vi "HEWH Build Draw Water States.vi"(8 "error in (no error)":errorcluster, 9 "Start Draw":bool, 10 "Full Cutout?":bool, 11 "Station":string) -> (0 "error out":errorcluster, 3 "result string":string)   [LabVIEW 2019]
uses:
  Type Definitions/HEWH Set Draw States.ctl
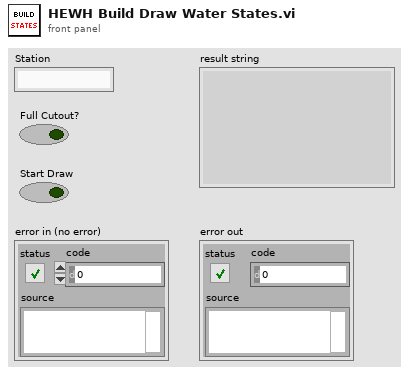
[diagram p1: front panel]
types:
  T1 = typedef "HEWH Set Draw States.ctl" = enum16{"Set Draw States", "Temperature Decline"}
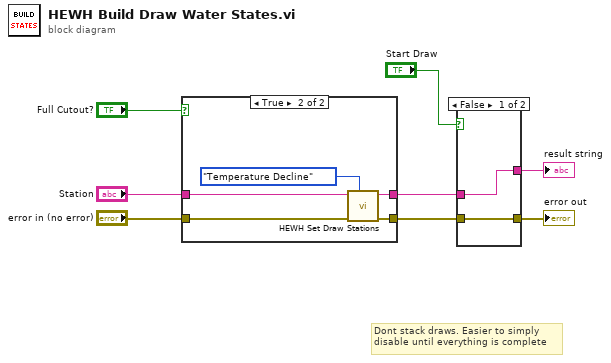
[diagram p0: block diagram]
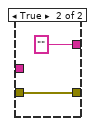
[diagram p2: hidden frame]
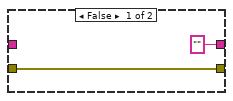
[diagram p3: hidden frame]
diagram:
  # "Dont stack draws. Easier to simply \ndisable until everything is complete"
  n1 = case shown="True" "Full Cutout?" {
    tunnel: ["" w15] -> w2
    tunnel: "error in (no error)" -> [w9 w13]
    tunnel: [w9 w12] -> w5
    tunnel: "Station" -> [_ w14]
    frame False {
    }
    frame True {
      n2 = call "HEWH Set Draw Stations.vi"("Draw States"=HEWH_Set_Draw_States."Temperature Decline", "Error In"=w13, "Station"=w14) -> ("Error Out"=w12:errorcluster, "result string"=w15:string)  [unwired: 7 in]
    }
  }
  n3 = case shown="False" "Start Draw" {
    tunnel: w2 -> [w17 _]
    tunnel: [w17 "" ("result string")] -> w4
    tunnel: w5 -> [w16 w18]
    tunnel: [w16 w18] -> w6
    frame False {
    }
    frame True {
    }
  }
  "error out" <- w6
  "result string" <- w4
